vi "TOML to tree Example.vi"() -> ()   [LabVIEW 2020]
doc: "This example demonstrates how to parse a TOML file"
uses:
  991fca34-f934-4be7-a00a-9118e7967e6b.vi
  lib/TOML to LabVIEW.vi
  lib/TOML.lvlib
panel:
  out "error out":errorcluster
  out "Parsed Data":T1 {"owner"."dob" format="%<%Y-%m-%d\n%H:%M:%S%3u%z>T"}
  out "TOML String":string
  in  "tree":string(tree)
  in  "TOML String":string="# This is a TOML document.\n\ntitle = \"TOML Example\"\n\n[owner]\nname = \"David Taylor\"\ndob = 1991-07-17T07:12:00-07:00 # First class dates\n\n[database]\nserver = \"192.168.1.1\"\nports = [ 8001, 8001, 8002 ]\nconnection_max = 5000\nenabled = true\n\n[servers]\n\n  # Indentation (tabs and/or spaces) is allowed but not required\n  [servers.alpha]\n  ip = \"10.0.0.1\"\n  dc = \"eqdc10\"\n\n  [servers.beta]\n  ip = \"10.0.0.2\"\n  dc = \"eqdc10\"\n\n[clients]\ndata = [ [\"gamma\", \"delta\"], [1, 2] ]\n\n# Line breaks are OK when inside arrays\nhosts = [\n  \"alpha\",\n  \"omega\"\n]\n\n#inline table\ninline_table = {one = 1, two = 2}\n\n[[array_of_tables]]\nmulti-line-string = \"\"\"\nline one\nline two\"\"\"\n\n[[array_of_tables]]\nmulti-line-literal-string = '''\nliteral strings allow special characters \\ unescaped\nline two'''"
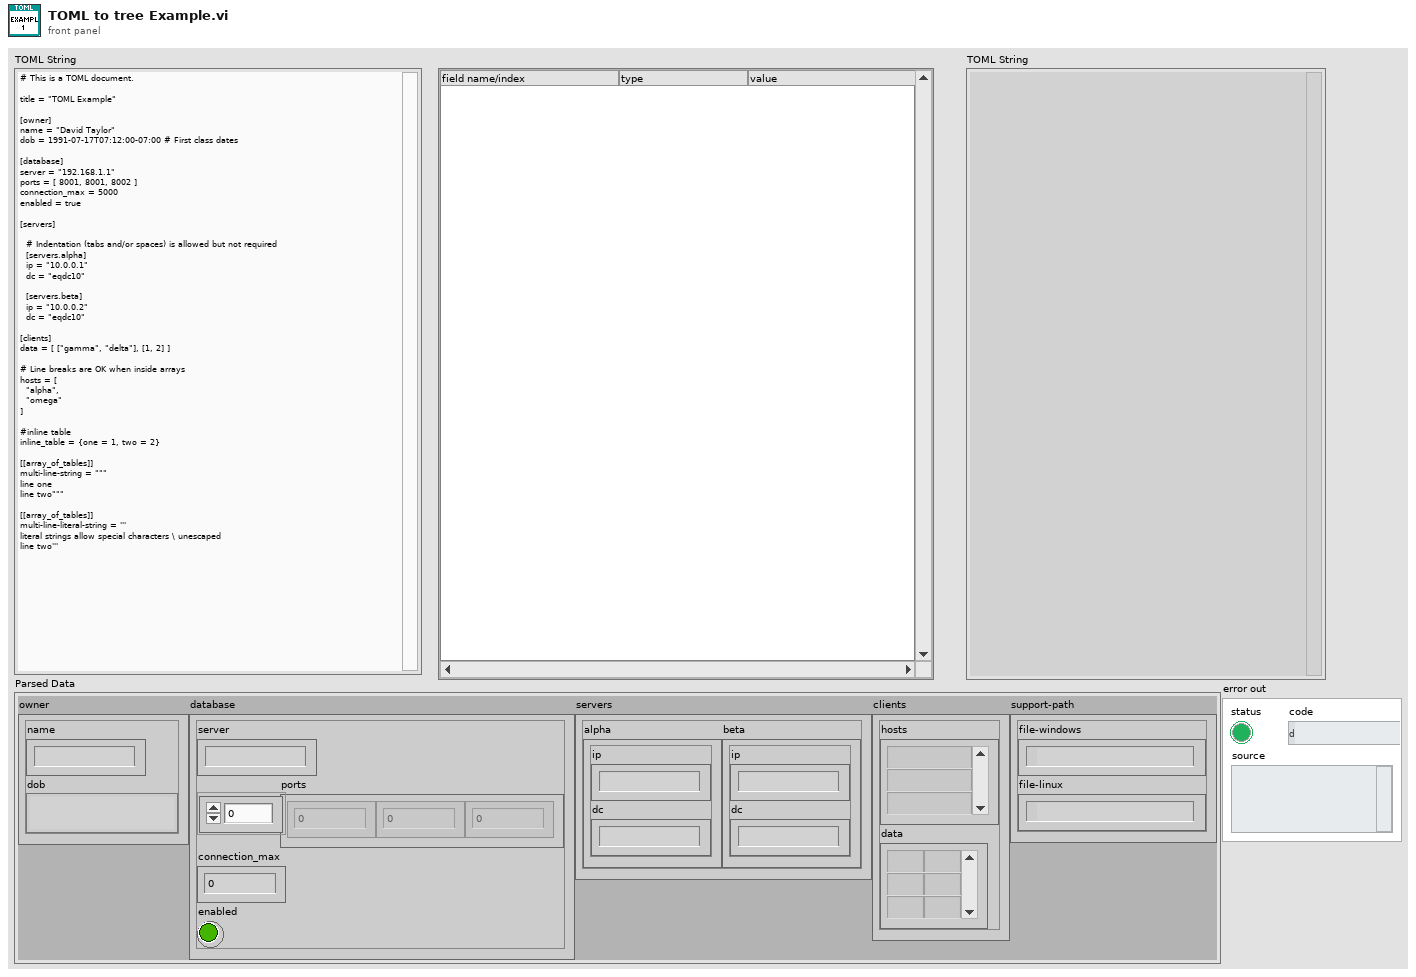
[diagram p1: front panel]
types:
  T1 = cluster{"owner":cluster{"name":string, "dob":timestamp}, "database":cluster{"server":string, "ports":u16[], "connection_max":dbl, "enabled":bool}, "servers":cluster{"alpha":cluster{"ip":string, "dc":string}, "beta":cluster{"ip":string, "dc":string}}, "clients":cluster{"hosts":string[], "data":string[][]}, "support-path":cluster{"file-windows":path, "file-linux":path}}
  T2 = typedef "TOML.lvlib/TOML Value.ctl" = cluster{"type":enum16{"Table", "Array", "String", "Integer", "Float", "Boolean", "Offset Date-Time", "Local Date-Time", "Local Date", "Local Time", "Path"}, "value":variant}
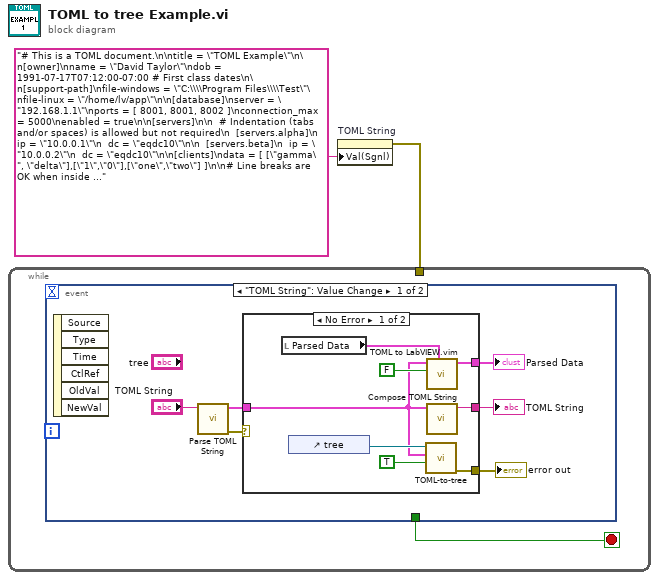
[diagram p0: block diagram]
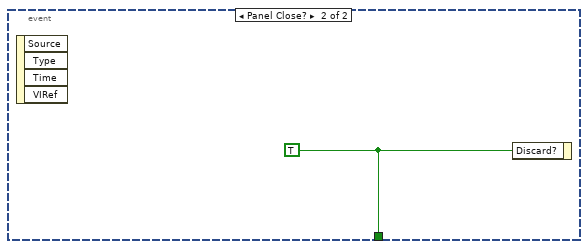
[diagram p3: hidden frame]
diagram:
  n1 = property on="TOML String" class="Str"("Val(Sgnl)"="# This is a TOML document.\n\ntitle = \"TOML Example\"\n\n[owner]\nname = \"David Taylor\"\ndob = 1991-07-17T07:12:00-07:00 # First class dates\n\n[support-path]\nfile-windows = \"C:\\\\Program Files\\\\Test\"\nfile-linux = \"/home/lv/app\"\n\n[database]\nserver = \"192.168.1.1\"\nports = [ 8001, 8001, 8002 ]\nconnection_max = 5000\nenabled = true\n\n[servers]\n\n  # Indentation (tabs and/or spaces) is allowed but not required\n  [servers.alpha]\n  ip = \"10.0.0.1\"\n  dc = \"eqdc10\"\n\n  [servers.beta]\n  ip = \"10.0.0.2\"\n  dc = \"eqdc10\"\n\n[clients]\ndata = [ [\"gamma\", \"delta\"],[\"1\",\"0\"],[\"one\",\"two\"] ]\n\n# Line breaks are OK when inside arrays\nhosts = [\n  \"alpha\",\n  \"omega\"\n]\n\n#inline table\ninline_table = {one = 1, two = 2}\n\n[[array_of_tables]]\nmulti-line-string = \"\"\"\nline one\nline two\"\"\"\n\n[[array_of_tables]]\nmulti-line-literal-string = '''\nliteral strings allow special characters \\ unescaped\nline two'''" ("TOML String")) -> (error out=w1:errorcluster)  [unwired: 2 in, 1 out]
  n2 = while {
    tunnel: w1 -> [_]
    stop <- w3 stop-if-true
    n3 = event shown="[0] \"TOML String\": Value Change" {
      selector: _ -> [_ _]
      dyn-events: _ -> [_ _]
      timeout: _ -> [_ _]
      tunnel: [_ w18] -> w3
      event "TOML String": Value Change {
        n4 = event-data() -> ()  [unwired: 1 in, 6 out]
        n5 = call "Parse TOML String.vi"("String"="TOML String") -> ("error out"=w9:errorcluster, "Value"=w7:T2)  [unwired: 9 in]
        n6 = case shown="No Error" w9 {
          tunnel: w7 -> [w10 _]
          tunnel: [w14 _] -> w6
          tunnel: [w15 _] -> w5
          tunnel: [w12 _] -> w4
          frame No Error {
            n7 = local read "Parsed Data"() -> (w17:T1)
            n8 = control-ref of="tree"() -> (w13:refnum<vi>)
            n9 = call "TOML-to-tree.vi"("purge"=TRUE, "value"=w10, "tree-control-ref"=w13) -> ("error out"=w12:errorcluster)  [unwired: 8 in]
            n10 = call "TOML to LabVIEW.vim"("datatype"=w17, "Error if missing element"=FALSE, "Value"=w10) -> ("LV Data"=w14:T1)  [unwired: 6 in, 2 out]
            n11 = call "Compose TOML String.vi"("Value"=w10) -> ("String"=w15:string)  [unwired: 9 in, 1 out]
          }
          frame Error {
          }
        }
        "Parsed Data" <- w6
        "TOML String" <- w5
        "error out" <- w4
      }
      event Panel Close? {
        w18 = TRUE
        n12 = event-data() -> ()  [unwired: 1 in, 4 out]
        n13 = event-data("Discard?"=w18) -> ()  [unwired: 1 in, 1 out]
      }
    }
  }
